vi "(SubVI) Slowly Go to Target PosiitonPI_YCC.vi"(4 "scan rate  (um/s)":dbl=2.0 format="%.3f", 5 "axis":u32=1, 6 "Target position (um)":dbl=50.0) -> (2 "Now position (um)":dbl)   [LabVIEW 2014]
panel:
  out "traveling time (s)":dbl
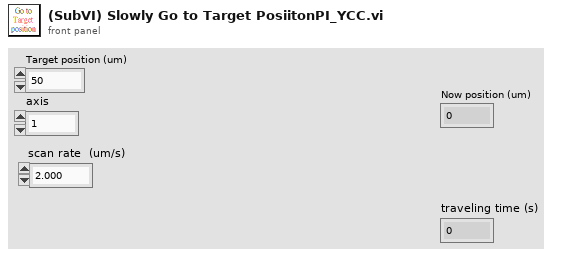
[diagram p1: front panel]
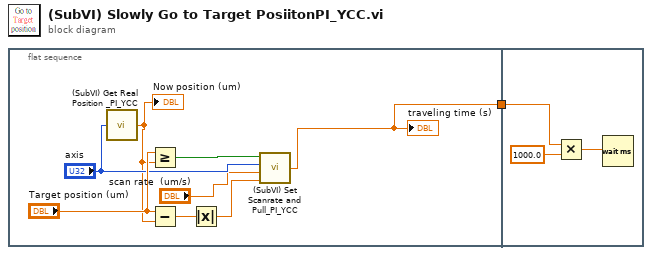
[diagram p0: block diagram]
diagram:
  n1 = flat-sequence {
    tunnel: [w3] -> w1
    tunnel: w1 -> [w10]
    frame #0 {
      n2 = call "(SubVI) Get Real Position _PI_YCC.vi"("Axis"="axis") -> ("Real Current Commanded position (um)"=w2:dbl)  [unwired: 4 in]
      "Now position (um)" <- w2
      n3 = Greater Or Equal?(x="Target position (um)", y=w2) -> (x >= y?=w9:bool)
      n4 = Subtract(x="Target position (um)", y=w2) -> (x-y=w7:dbl)
      n5 = Absolute Value(x=w7) -> (abs(x)=w6:dbl)
      n6 = call "(SubVI) Set Scanrate and Pull_PI_YCC.vi"("toward+ ?\nT=+, F=-"=w9, "axis"="axis", "scan rate  (um/s)"="scan rate  (um/s)", "range  (um)"=w6) -> ("Traveling time (s)"=w3:dbl)  [unwired: 3 in, 1 out]
      "traveling time (s)" <- w3
    }
    frame #1 {
      n7 = Multiply(x=w10, y=1000.0) -> (x*y=w12:dbl)
      n8 = Wait (ms)(milliseconds to wait=w12) -> ()  [unwired: 1 out]
    }
  }
